vi "PID Deadband Timeout.vi"(10 "Time to Wait":i32=10, 11 "In deadband range?":bool) -> (3 "Deadband Timed-out":bool)   [LabVIEW 2014]
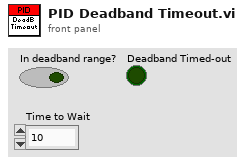
[diagram p1: front panel]
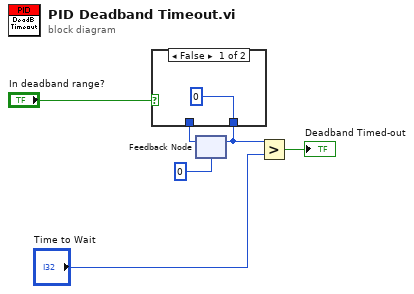
[diagram p0: block diagram]
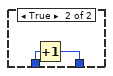
[diagram p2: hidden frame]
diagram:
  n1 = feedback #1(0) -> (w3:i32)
  n2 = case shown="False" "In deadband range?" {
    tunnel: [0 w9] -> w4
    tunnel: w3 -> [_ w8]
    frame False {
    }
    frame True {
      n3 = Increment(x=w8) -> (x+1=w9:i32)
    }
  }
  n4 = feedback-in #1(w4) -> ()
  n5 = Greater?(x=w4, y="Time to Wait") -> (0:→"Deadband Timed-out":bool)
